vi "xiLIB - GetGPIStates.vi"(8 "error in (no error)":errorcluster, 11 "xiCam In":refnum<k24>) -> (0 "error out":errorcluster, 3 "xiCam Out":refnum<k24>, 4 "GPI_States[] - NUM":cluster{"GPI_INDEX":i32, "GPI_MODE":T1}[](array[cluster]), 6 "GPI_States[] - STR":cluster{"GPI_INDEX":string, "GPI_MODE":string}[](array[cluster]))   [LabVIEW 2018]
doc: "Returns the current GPI States of Camera."
uses:
  D:/codes labview/VisionLibrariesXimea/xiLib/xiLIB_64bit/xiLIB/xiCamLib/API/x64/xiApi.NETX64.dll
  API/x64/xiApi.NETX64.dll
  xiCam/PRM/GPI_MODE/GPI_MODE.ctl
  xiCam/PRM/PRM/PRM_v2.ctl
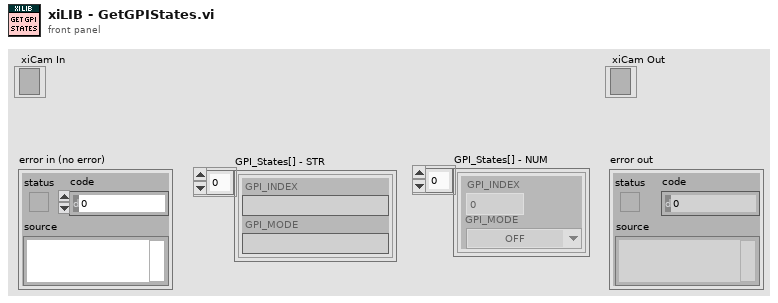
[diagram p1: front panel]
types:
  T1 = typedef "GPI_MODE.ctl" = enum16{"OFF", "TRIGGER", "EXT_EVENT"}
  T2 = typedef "PRM_v2.ctl" = enum16{"ACQ_BUFFER_SIZE", "ACQ_FRAME_BURST_COUNT", "ACQ_TIMING_MODE", "ACQ_TRANSPORT_BUFFER_SIZE", "AE_MAX_LIMIT", "AEAG", "AEAG_LEVEL", "API_VERSION", "AG_MAX_LIMIT", "APPLY_CMS", "AUTO_BANDWIDTH_CALCULATION", "AUTO_WB", "AVAILABLE_BANDWIDTH", "AVAILABLE_BANDWIDTH_MAX", "AVAILABLE_BANDWIDTH_MIN", "BPC", "BUFFER_POLICY", "BUFFERS_QUEUE_SIZE", "CC_MATRIX_00", "CC_MATRIX_01", "CC_MATRIX_02", "CC_MATRIX_03", "CC_MATRIX_10", "CC_MATRIX_11", "CC_MATRIX_12", "CC_MATRIX_13", "CC_MATRIX_20", "CC_MATRIX_21", "CC_MATRIX_22", "CC_MATRIX_23", "CC_MATRIX_30", "CC_MATRIX_31", "CC_MATRIX_32", "CC_MATRIX_33", "CHIP_TEMP", "CMS", "COLOR_FILTER_ARRAY", "COOLING", "DEBOUNCE_EN", "DEBOUNCE_POL", "DEBOUNCE_T0", "DEBOUNCE_T1", "DEBUG_LEVEL", "DEFAULT_CC_MATRIX", "DEVICE_INSTANCE_PATH", "DEVICE_MODEL_ID", "DEVICE_NAME", "DEVICE_SN", "DEVICE_TYPE", "DEVICE_USER_ID", "DOWNSAMPLING", "DOWNSAMPLING_MAX", "DOWNSAMPLING_MIN", "DOWNSAMPLING_TYPE", "DRV_VERSION", "EXP_PRIORITY", "EXPOSURE", "EXPOSURE_DIRECT_UPDATE", "EXPOSURE_MAX", "EXPOSURE_MIN", "FFS_FILE_NAME", "FPGA1_VERSION", "FRAMERATE", "FRAMERATE_MAX", "FRAMERATE_MIN", "FREE_FFS_SIZE", "GAIN", "GAIN_DIRECT_UPDATE", "GAIN_MAX", "GAIN_MIN", "GAMMAC", "GAMMAY", "GPI_LEVEL", "GPI_MODE", "GPI_SELECTOR", "GPI_SELECTOR_MAX", "GPI_SELECTOR_MIN", "GPO_MODE", "GPO_SELECTOR", "GPO_SELECTOR_MAX", "GPO_SELECTOR_MIN", "HDR", "HDR_T1", "HDR_T2", "HEIGHT", "HEIGHT_MAX", "HEIGHT_MIN", "HOUSE_TEMP", "IMAGE_DATA_FORMAT", "IMAGE_IS_COLOR", "INPUT_CMS_PROFILE", "IS_COOLED", "IS_DEVICE_EXIST", "KNEEPOINT1", "KNEEPOINT2", "LED_MODE", "LED_SELECTOR", "LED_SELECTOR_MAX", "LED_SELECTOR_MIN", "LIMIT_BANDWIDTH", "LIMIT_BANDWIDTH_MAX", "LIMIT_BANDWIDTH_MIN", "LUT_EN", "LUT_INDEX", "LUT_INDEX_MAX", "LUT_INDEX_MIN", "LUT_VALUE", "LUT_VALUE_MAX", "LUT_VALUE_MIN", "MANUAL_WB", "MCU1_VERSION", "MCU2_VERSION", "OFFSET_X", "OFFSET_X_MAX", "OFFSET_X_MIN", "OFFSET_Y", "OFFSET_Y_MAX", "OFFSET_Y_MIN", "OUTPUT_CMS_PROFILE", "OUTPUT_DATA_BIT_DEPTH", "OUTPUT_DATA_PACKING", "READ_FILE_FFS", "RECENT_FRAME", "SENSOR_DATA_BIT_DEPTH", "SENSOR_MODE", "SENSOR_TAPS", "SHARPNESS", "SHUTTER_TYPE", "TARGET_TEMP", "TRG_DELAY", "TRG_SELECTOR", "TRG_SOFTWARE", "TRG_SOURCE", "USED_FFS_SIZE", "WB_KB", "WB_KG", "WB_KR", "WIDTH", "WIDTH_MAX", "WIDTH_MIN", "WRITE_FILE_FFS", "ACQ_BUFFER_SIZE_UNIT", "ACQ_TRANSPORT_BUFFER_COMMIT", "AEAG_ROI_HEIGHT", "AEAG_ROI_OFFSET_X", "AEAG_ROU_OFFSET_Y", "AEAG_ROI_WIDTH", "API_CONTEXT_LIST", "BINNING_HORIZONTAL", "BINNING_SELECTOR", "BINNING_VERTICAL", "COLUMN_FPN_CORRECTION", "COUNTER_SELECTOR", "COUNTER_VALUE", "DECIMATION_HORIZONTAL", "DECIMATION_SELECTOR", "DECIMATION_VERTICAL", "DEVICE_ID", "DEVICE_LOCATION_PATH", "DEVICE_MANIFEST", "DEVICE_RESET", "DEVICE_SENS_SN", "EXPOSURE_BURST_COUNT", "FFS_ACCESS_KEY", "GAIN_SELECTOR", "HW_REVISION", "IMAGE_BLACK_LEVEL", "IMAGE_DATA_BIT_DEPTH", "IMAGE_DATA_FORMAT_RGB32_ALPHA", "IMAGE_PAYLOAD_SIZE", "LENS_APERTURE_VALUE", "LENS_FEATURE", "LENS_FEATURE_SELECTOR", "LENS_FOCAL_LENGTH", "LENS_FOCUS_DISTANCE", "LENS_FOCUS_MOVE", "LENS_FOCUS_MOVEMENT_VALUE", "LENS_MODE", "OUTPUT_DATA_PACKING_TYPE", "SENSOR_CLOCK_FREQ_HZ", "SENSOR_CLOCK_FREQ_INDEX", "SENSOR_FEATURE_SELECTOR", "SENSOR_FEATURE_VALUE", "SENSOR_OUTPUT_CHANNEL_COUNT", "TRANSPORT_PIXEL_FORMAT", "TS_RST_MODE", "TS_RST_SOURCE"}
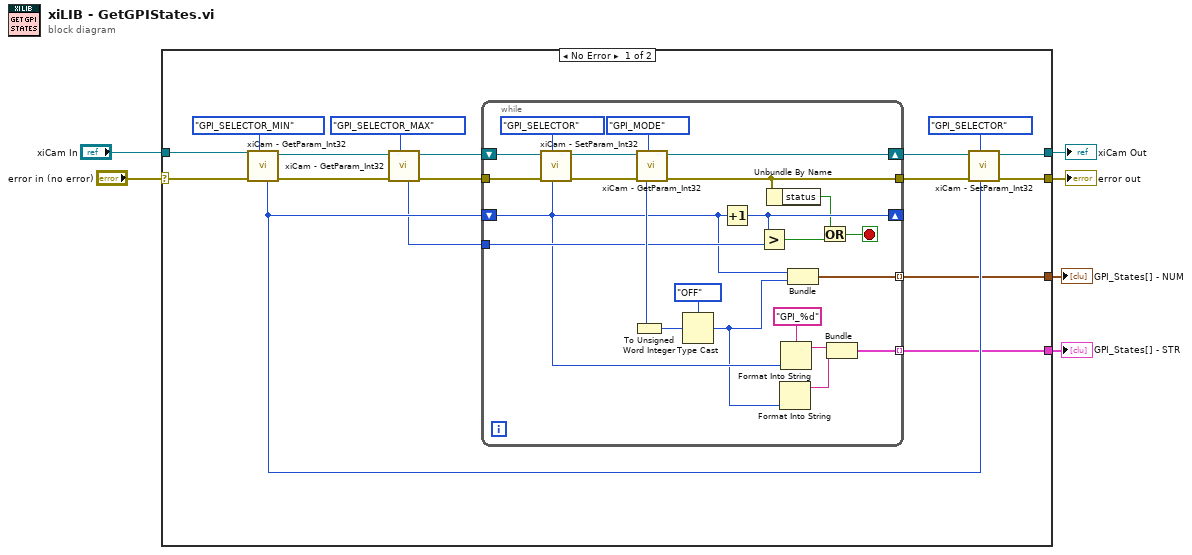
[diagram p0: block diagram]
diagram:
  n1 = case shown="No Error" "error in (no error)" {
    selector: "error in (no error)" -> [w21 w47]
    tunnel: "xiCam In" -> [w23 w48]
    tunnel: [w12 w48] -> w4
    tunnel: [w11 w47] -> w3
    tunnel: [w8 _] -> w2
    tunnel: [w7 _] -> w1
    frame No Error {
      n2 = call "xiCam - GetParam_Int32.vi"("PRM"=PRM_v2."GPI_SELECTOR_MIN", "error in (no error)"=w21, "xiCam In"=w23) -> ("error out"=w18:errorcluster, "xiCam Out"=w19:refnum<k24>, "Int32_Value"=w10:i32)  [unwired: 6 in]
      n3 = call "xiCam - GetParam_Int32.vi"("PRM"=PRM_v2."GPI_SELECTOR_MAX", "error in (no error)"=w18, "xiCam In"=w19) -> ("error out"=w16:errorcluster, "xiCam Out"=w17:refnum<k24>, "Int32_Value"=w9:i32)  [unwired: 6 in]
      n4 = while {
        tunnel: w16 -> [w44]
        shift-right: [w37] -> _
        shift-left: w10 -> [w29]
        shift-right: [w40] -> w14
        shift-left: w17 -> [w45]
        tunnel: [w35] -> w13
        tunnel: w9 -> [w38]
        tunnel: [w32] -> w8 mode=indexing
        tunnel: [w24] -> w7 mode=indexing
        stop <- w31 stop-if-true
        n5 = call "xiCam - SetParam_Int32.vi"("Int32_Value"=w29, "PRM"=PRM_v2."GPI_SELECTOR", "error in (no error)"=w44, "xiCam In"=w45) -> ("error out"=w41:errorcluster, "xiCam Out"=w42:refnum<k24>)  [unwired: 6 in]
        n6 = call "xiCam - GetParam_Int32.vi"("PRM"=PRM_v2."GPI_MODE", "error in (no error)"=w41, "xiCam In"=w42) -> ("error out"=w35:errorcluster, "xiCam Out"=w40:refnum<k24>, "Int32_Value"=w39:i32)  [unwired: 6 in]
        n7 = To Unsigned Word Integer(number=w39) -> (unsigned 16bit integer=w33:u16)
        n8 = Type Cast(type=GPI_MODE."OFF" ("GPI_MODE"), x=w33) -> (*(type *) &x=w27:T1)
        n9 = Increment(x=w29) -> (x+1=w37:i32)
        n10 = Greater?(x=w37, y=w38) -> (0:w36:bool)
        n11 = Unbundle By Name(w35) -> ("status"=w34:bool)
        n12 = Format Into String(w27) -> (resulting string=w25:string)  [unwired: 3 in, 1 out]
        n13 = Format Into String(format string="GPI_%d", w29) -> (resulting string=w26:string)  [unwired: 2 in, 1 out]
        n14 = Bundle("Int32_Value"=w29, "GPI_MODE"=w27) -> (w32:cluster{"Int32_Value":i32, "GPI_MODE":T1})  [unwired: 1 in]
        n15 = Or(x=w34, y=w36) -> (x .or. y?=w31:bool)
        n16 = Bundle(w26, w25) -> (w24:cluster{string, string})  [unwired: 1 in]
      }
      n17 = call "xiCam - SetParam_Int32.vi"("Int32_Value"=w10, "PRM"=PRM_v2."GPI_SELECTOR", "error in (no error)"=w13, "xiCam In"=w14) -> ("error out"=w11:errorcluster, "xiCam Out"=w12:refnum<k24>)  [unwired: 6 in]
    }
    frame Error {
    }
  }
  "error out" <- w3
  "xiCam Out" <- w4
  "GPI_States[] - NUM" <- w2
  "GPI_States[] - STR" <- w1
